vi "BuyStock.vi"(8 "error in (no error)":errorcluster, 10 "Stock.lvclass":refnum<class "Stock.lvclass">, 11 "BuyStock in":refnum<class "BuyStock.lvclass">) -> (0 "error out":errorcluster, 3 "BuyStock out":refnum<class "BuyStock.lvclass">)   [LabVIEW 2017, in "BuyStock.lvclass"]
uses:
  BuyStock.lvclass
  Stock Class/Stock.lvclass
  BuyStock.lvclass/BuyStock.ctl
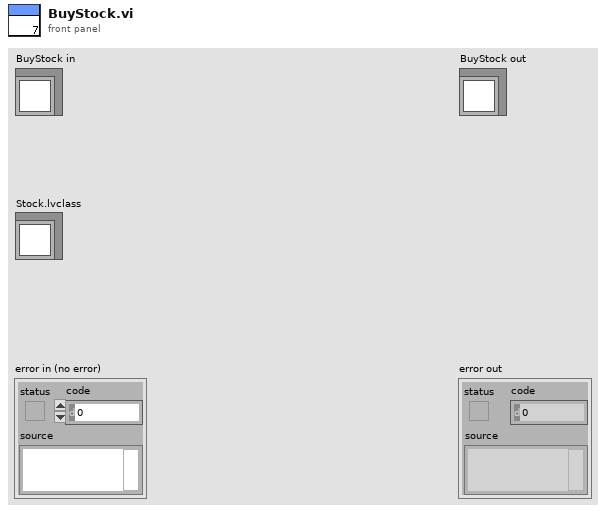
[diagram p1: front panel]
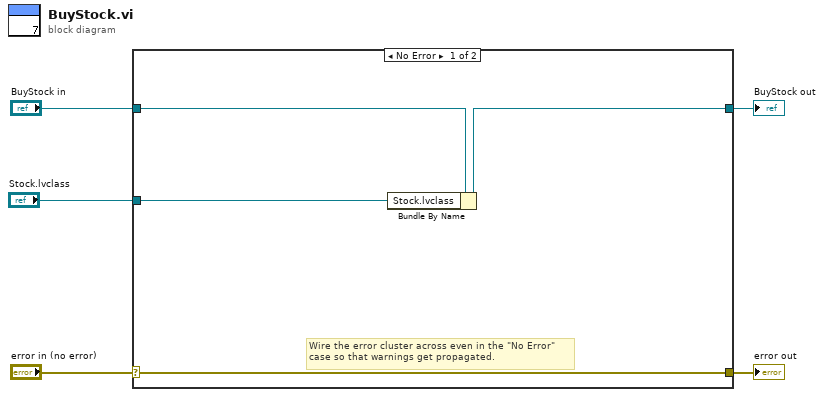
[diagram p0: block diagram]
diagram:
  n1 = case shown="No Error" "error in (no error)" {
    selector: "error in (no error)" -> [w8 w11]
    tunnel: [w8 w11] -> w4
    tunnel: [w7 w10] -> w2
    tunnel: "BuyStock in" -> [w9 w10]
    tunnel: "Stock.lvclass" -> [w6 _]
    frame No Error {
      # "Wire the error cluster across even in the \"No Error\"\ncase so that warnings get propagated."
      n2 = Bundle By Name(cluster=w9, "Stock.lvclass"=w6) -> (w7:refnum<class "BuyStock.lvclass">)
    }
    frame Error {
    }
  }
  "error out" <- w4
  "BuyStock out" <- w2
